vi "Navigating Structures.vi"() -> ()   [LabVIEW 2019]
doc: "This VI uses navigation techniques to determine whether a target VI contains any Case structures whose case selector is wired to a constant. \n\nThe Detailed Help explains how this example illustrates a general procedure for navigating across a structure in a target VI."
uses:
  <vilib>/Utility/traverseref.llb/TRef TravTarget.ctl
  <vilib>/Utility/traverseref.llb/VI Scripting - Traverse.lvlib
panel:
  out "Number of Case Structures Wired To Constant":i32
  # "Select Help>>Show Context Help and move the cursor over the VI icon to display help for this VI.\n\nBefore you start: Open the Detailed Help for this example to display the Navigating across a Structure Using VI Scripting topic in the  LabVIEW Help. That topic provides additional details about how this example illustrates the general procedure for navigating across a structure in a target VI.\n\nThis scripting VI demonstrates how to navigate across Case structures in a target VI to determine whether the Case Structures have a constant wired to their case selector."
  # "Overview: Demonstrates the use of VI Scripting to programmatically inspect a diagram containing structures (loops, case structures, event structures, etc.).\nInstructions:\nRun the VI. The indicator below will display the number of case structures in Test - Navigating Structures Target.vi that have a constant wired to their case selectors."
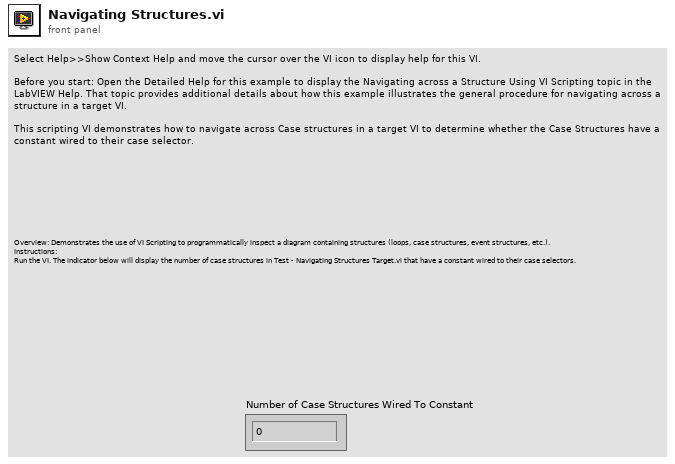
[diagram p1: front panel]
types:
  T1 = typedef "TRef TravTarget.ctl" = enum16{"FP", "BD", "Other"}
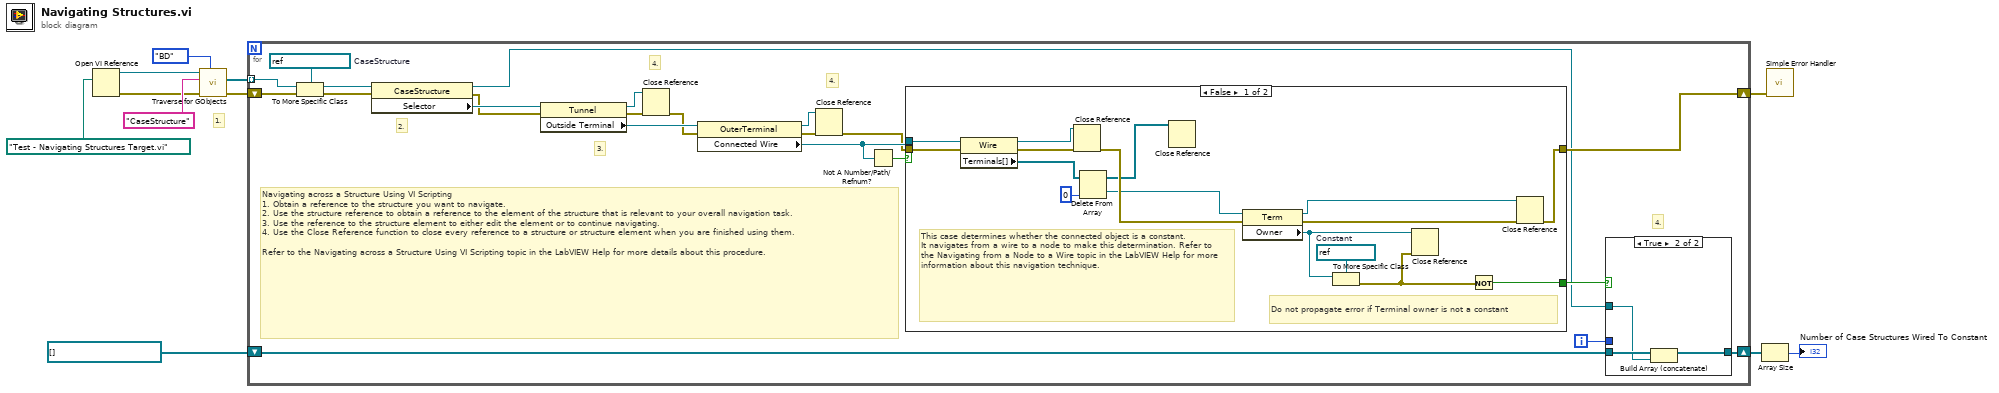
[diagram p0: block diagram]
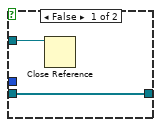
[diagram p3: hidden frame]
diagram:
  # "1."
  n1 = Open VI Reference(vi path=path "Test - Navigating Structures Target.vi" ("VI Path")) -> (vi reference=w5:refnum<vi>, error out=w4:errorcluster)  [unwired: 5 in]
  n2 = call <vilib>:"Traverse for GObjects.vi"("Traverse Target"=TRef_TravTarget."BD", "error in (no error)"=w4, "Class Name"="CaseStructure", "VI Refnum"=w5) -> ("error out"=w8:errorcluster, "References"=w1:refnum<vi>[])  [unwired: 4 in, 2 out]
  n3 = for {
    shift-right: [w30] -> w10
    shift-left: refnum<vi>[] [] ("Case Structures Wired To Constant") -> [w31]
    tunnel: w1 -> [w28] mode=indexing
    shift-right: [w16] -> w2
    shift-left: w8 -> [w14]
    i -> [w23]
    w32 = refnum<vi> refnum  # CaseStructure
    # "4."
    # "Navigating across a Structure Using VI Scripting\n1. Obtain a reference to the structure you want to navigate.\n2. Use the structure reference to obtain a reference to the element of the structure that is relevant to your overall navigation task.\n3. Use the reference to the structure element to either edit the element or to continue navigating.\n4. Use the Close Reference function to close every reference to a structure or structure element when you are finished using them.\n\nRefer to the Navigating across a Structure Using VI Scripting topic in the LabVIEW Help for more details about this procedure."
    # "4."
    # "4."
    # "3."
    # "2."
    n4 = To More Specific Class(target class=w32, reference=w28, error in=w14) -> (specific class reference=w15:refnum<vi>, error out=w33:errorcluster)
    n5 = property on="Property Node" class="CaseStructure"(reference=w15, error in=w33) -> (reference out=w13:refnum<vi>, error out=w12:errorcluster, "Selector"=w27:refnum<vi>)
    n6 = property on="Property Node" class="Tunnel"(reference=w27, error in=w12) -> (reference out=w21:refnum<vi>, error out=w22:errorcluster, "Outside Terminal"=w26:refnum<vi>)
    n7 = Close Reference(reference=w21, error in (no error)=w22) -> (error out=w20:errorcluster)
    n8 = property on="Property Node" class="OuterTerminal"(reference=w26, error in=w20) -> (reference out=w18:refnum<vi>, error out=w19:errorcluster, "Connected Wire"=w25:refnum<vi>)
    n9 = Close Reference(reference=w18, error in (no error)=w19) -> (error out=w17:errorcluster)
    n10 = Not A Number/Path/Refnum?(number/path/refnum=w25) -> (NaN/Path/Refnum?=w24:bool)
    n11 = case shown="False" w24 {
      tunnel: [w40 w50] -> w16
      tunnel: [w47 _] -> w29
      tunnel: w25 -> [w49 _]
      tunnel: w17 -> [w48 w50]
      frame False {
        w38 = refnum<vi> refnum  # Constant
        # "Do not propagate error if Terminal owner is not a constant"
        # "This case determines whether the connected object is a constant.\nIt navigates from a wire to a node to make this determination. Refer to the Navigating from a Node to a Wire topic in the LabVIEW Help for more information about this navigation technique."
        n12 = property class="Wire"(reference=w49, error in=w48) -> (reference out=w45:refnum<vi>, error out=w46:errorcluster, "Terminals[]"=w43:refnum<vi>[])
        n13 = Close Reference(reference=w45, error in (no error)=w46) -> (error out=w44:errorcluster)
        n14 = Delete From Array(array=w43, index=0) -> (deleted portion=w39:refnum<vi>, array with subset deleted=w41:refnum<vi>[])  [unwired: 1 in]
        n15 = Close Reference(reference=w41) -> ()  [unwired: 1 in, 1 out]
        n16 = property class="Term"(reference=w39, error in=w44) -> (reference out=w36:refnum<vi>, error out=w35:errorcluster, "Owner"=w37:refnum<vi>)
        n17 = To More Specific Class(target class=w38, reference=w37) -> (error out=w34:errorcluster)  [unwired: 1 in, 1 out]
        n18 = Close Reference(reference=w37, error in (no error)=w34) -> ()  [unwired: 1 out]
        n19 = Not(x=w34) -> (.not. x?=w47:bool)
        n20 = Close Reference(reference=w36, error in (no error)=w35) -> (error out=w40:errorcluster)
      }
      frame True {
        # "Selector terminal unwired"
      }
    }
    n21 = case shown="True" w29 {
      tunnel: w31 -> [w52 w55]
      tunnel: [w52 w54] -> w30
      tunnel: w23 -> [_ _]
      tunnel: w13 -> [w51 w53]
      frame False {
        n22 = Close Reference(reference=w51) -> ()  [unwired: 1 in, 1 out]
      }
      frame True {
        n23 = Build Array (concatenate)(w55, w53) -> (w54:refnum<vi>[])
      }
    }
  }
  n24 = Array Size(array=w10) -> (size(s)=→"Number of Case Structures Wired To Constant":i32)
  n25 = call <vilib>:"Simple Error Handler.vi"("error in (no error)"=w2) -> ()  [unwired: 4 in, 5 out]
